vi "RetrieveData.vi"(8 "error in (no error)":errorcluster, 9 "pointsToRetrieve":i32, 11 "controller in":refnum<k24>) -> (0 "error out":errorcluster, 2 "Data Out":refnum<k24>, 3 "controller out":refnum<k24>)   [LabVIEW 2020, in "Aerotech.lvlib"]
uses:
  Aerotech.lvlib
  C:/Program Files (x86)/Aerotech/A3200/LabVIEW/2010/Bin/Aerotech.A3200.dll
  Program Files (x86)/Aerotech/A3200/LabVIEW/2010/Bin/Aerotech.A3200.dll
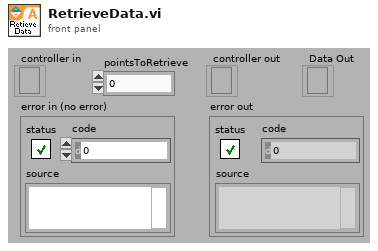
[diagram p1: front panel]
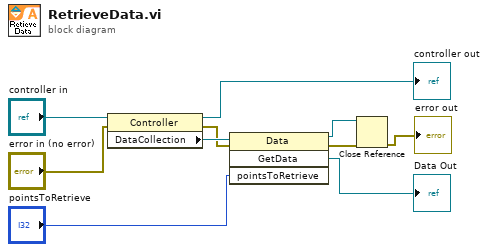
[diagram p0: block diagram]
diagram:
  n1 = property class="Controller"(reference="controller in", error in="error in (no error)") -> (reference out=→"controller out":refnum<k24>, error out=w7:errorcluster, "DataCollection"=w8:refnum<k24>)
  n2 = invoke class="Data" method="GetData"(reference=w8, error in=w7, "pointsToRetrieve"="pointsToRetrieve") -> (reference out=w4:refnum<k24>, error out=w2:errorcluster, "GetData"=→"Data Out":refnum<k24>)  [unwired: 1 in, 1 out]
  n3 = Close Reference(reference=w4, error in (no error)=w2) -> (error out=→"error out":errorcluster)
